vi "Export Config UI.vi"(10 "Config":T1) -> ()   [LabVIEW 2020, in "VolatusGUI.lvlib" / "Historian Charting Manager.lvclass"]
uses:
  Historian Charting Manager.lvclass
  JSON Charting Config.ctl
  JSON Chart Group.ctl
  JSON Plot Group.ctl
  JSON Plot Config.ctl
  Export State.ctl
  lv-tree-tools/Tree Map/Tree Map/Extra Entry Info.ctl
  7dad0396-1ecd-452e-bf08-d6d811beb585.vi
  <vilib>/JDP Science/JSONtext/Variant to JSON Text.vi
  <vilib>/JDP Science/JSONtext/LVClass Serializer/JSONtext LVClass Serializer.lvclass
  Historian Charting Manager.lvclass/Historian Charting Manager.ctl
  lv-tree-tools/Tree Map/Tree Map/Tree Map.lvclass
  VolatusGUI.lvlib
panel:
  in  "Cancel":bool
  in  "Accept":bool
  in  "Plot Groups":string(tree)
  in  "Chart Groups":string(tree)
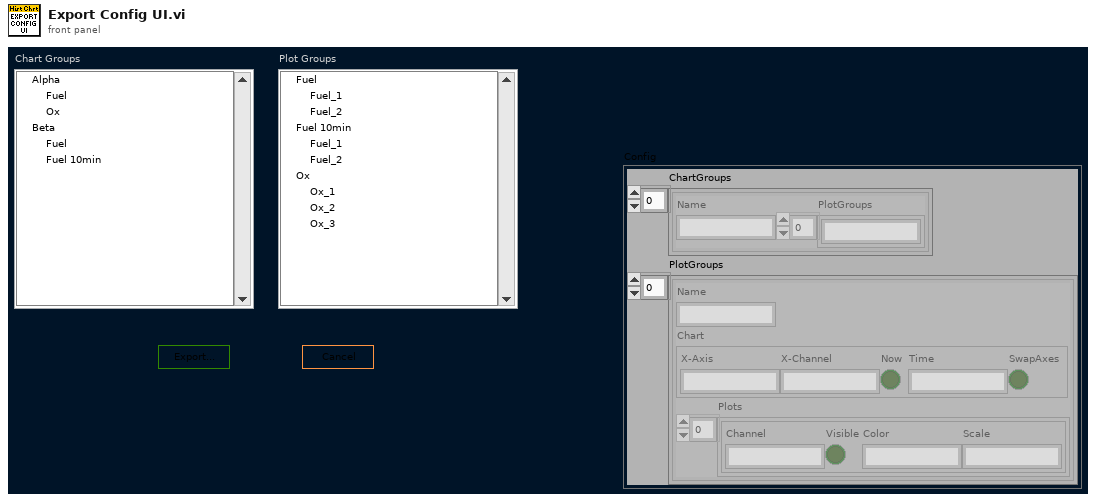
[diagram p1: front panel]
types:
  T1 = typedef "VolatusGUI.lvlib/JSON Charting Config.ctl" = cluster{"ChartGroups":T2[], "PlotGroups":T3[]}
  T2 = typedef "VolatusGUI.lvlib/JSON Chart Group.ctl" = cluster{"Name":string, "PlotGroups":string[]}
  T3 = typedef "VolatusGUI.lvlib/JSON Plot Group.ctl" = cluster{"Name":string, "Chart":cluster{"X-Axis":string, "X-Channel":string, "Now":bool, "Time":string, "SwapAxes":bool}, "Plots":T4[]}
  T4 = typedef "VolatusGUI.lvlib/JSON Plot Config.ctl" = cluster{"Channel":string, "Visible":bool, "Color":string, "Scale":string}
  T5 = typedef "VolatusGUI.lvlib/Historian Charting Manager.lvclass/Export State.ctl" = enum16{"Init", "Select", "Write"}
  T6 = typedef "Tree Map.lvlib/Tree Map.lvclass/Extra Entry Info.ctl" = cluster{"BG Color":u32, "Symbol":i32}
  T7 = enum32{"Invalid", "Standard", "Closed", "Hidden", "Minimized", "Maximized"}
  T8 = typedef "LVPoint32TypeDef.ctl" = cluster{"Horizontal":i32, "Vertical":i32}
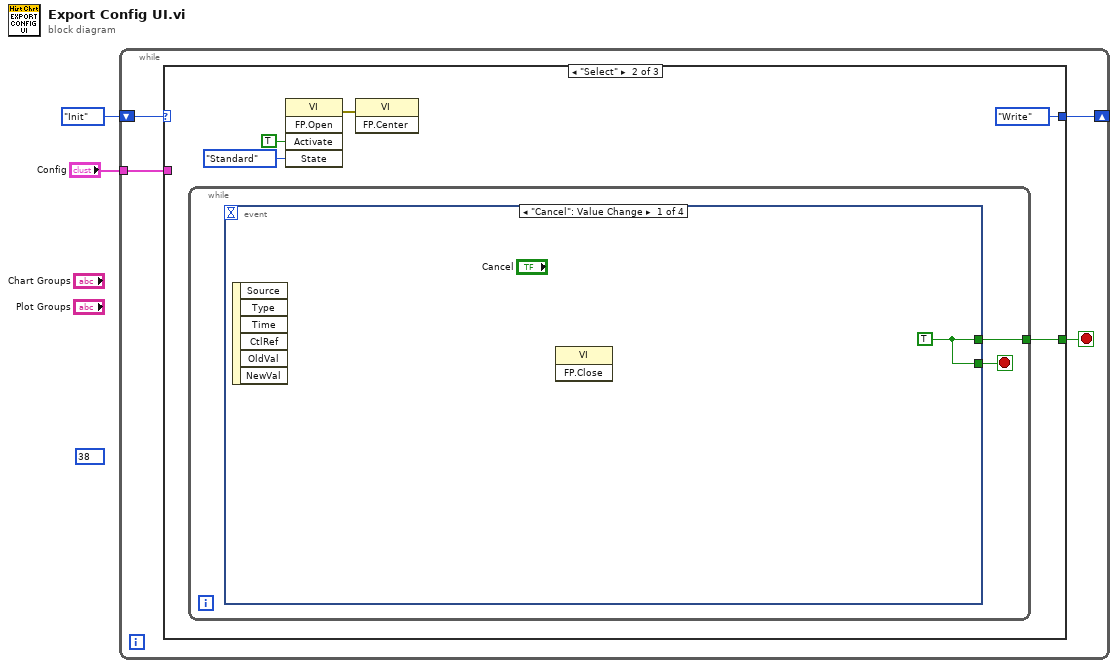
[diagram p0: block diagram]
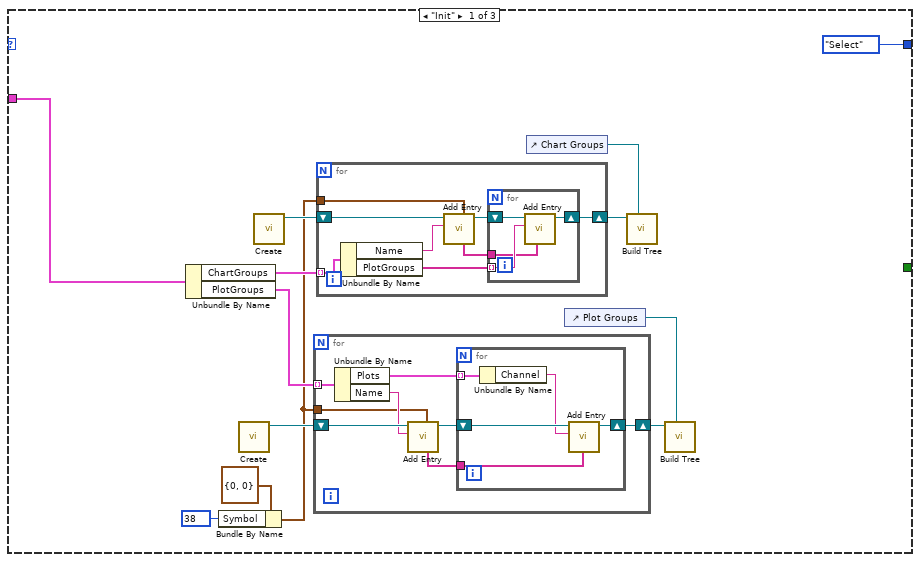
[diagram p2: hidden frame]
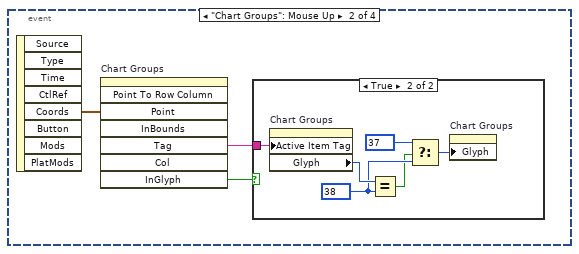
[diagram p3: hidden frame]
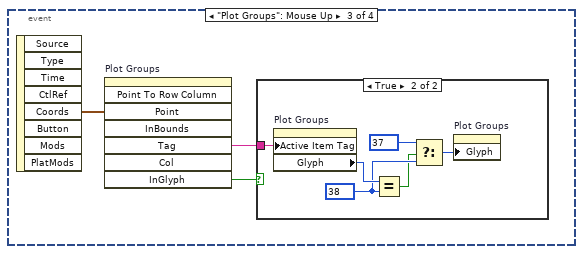
[diagram p5: hidden frame]
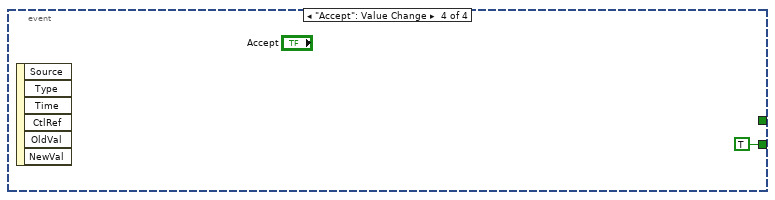
[diagram p7: hidden frame]
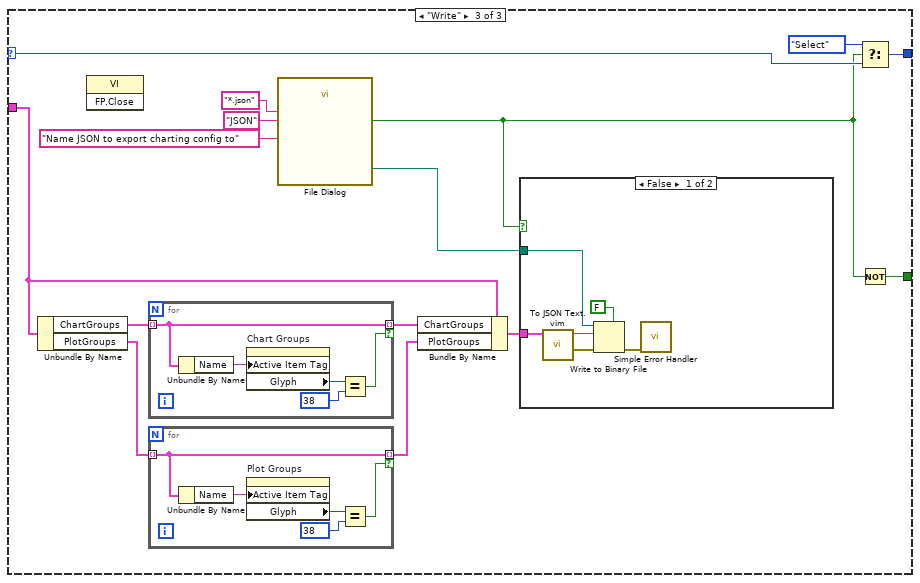
[diagram p8: hidden frame]
diagram:
  (unwired) 38
  n1 = while {
    shift-right: [w5] -> _
    shift-left: Export_State."Init" ("Export State") -> [w6]
    tunnel: "Config" -> [w4]
    stop <- w3 stop-if-true
    n2 = case shown="\"Select\"" w6 {
      selector: w6 -> [_ _ w81]
      tunnel: [Export_State."Select" ("Export State") Export_State."Write" ("Export State") w80] -> w5
      tunnel: w4 -> [w18 _ w74]
      tunnel: [_ w48 w82] -> w3
      frame "Init" {
        n3 = Unbundle By Name(w18) -> ("ChartGroups"=w17:T2[], "PlotGroups"=w13:T3[])
        n4 = Bundle By Name(cluster=T6 {"BG Color"=0, "Symbol"=0} ("Extra Info"), "Symbol"=38) -> (w7:T6)
        n5 = call "Create.vi"() -> ("Tree Map out"=w12:refnum<class "Tree Map.lvclass">)  [unwired: 10 in, 1 out]
        n6 = call "Create.vi"() -> ("Tree Map out"=w16:refnum<class "Tree Map.lvclass">)  [unwired: 10 in, 1 out]
        n7 = for {
          tunnel: w13 -> [w27] mode=indexing
          shift-right: [w21] -> w11
          shift-left: w12 -> [w26]
          tunnel: w7 -> [w20]
          n8 = Unbundle By Name(w27) -> ("Plots"=w23:T4[], "Name"=w25:string)
          n9 = call "Add Entry.vi"("Extra Info"=w20, "Name"=w25, "Tree Map in"=w26) -> ("Tree Map out"=w24:refnum<class "Tree Map.lvclass">, "Hierarchy"=w22:string[])  [unwired: 6 in, 1 out]
          n10 = for {
            shift-right: [w28] -> w21
            shift-left: w24 -> [w31]
            tunnel: w23 -> [w32] mode=indexing
            tunnel: w22 -> [w29]
            n11 = Unbundle By Name(w32) -> ("Channel"=w30:string)
            n12 = call "Add Entry.vi"("Parent (None)"=w29, "Name"=w30, "Tree Map in"=w31) -> ("Tree Map out"=w28:refnum<class "Tree Map.lvclass">)  [unwired: 6 in, 2 out]
          }
        }
        n13 = for {
          tunnel: w17 -> [w40] mode=indexing
          shift-right: [w34] -> w15
          shift-left: w16 -> [w39]
          tunnel: w7 -> [w33]
          n14 = Unbundle By Name(w40) -> ("Name"=w38:string, "PlotGroups"=w36:string[])
          n15 = call "Add Entry.vi"("Extra Info"=w33, "Name"=w38, "Tree Map in"=w39) -> ("Tree Map out"=w37:refnum<class "Tree Map.lvclass">, "Hierarchy"=w35:string[])  [unwired: 6 in, 1 out]
          n16 = for {
            shift-right: [w41] -> w34
            shift-left: w37 -> [w44]
            tunnel: w36 -> [w43] mode=indexing
            tunnel: w35 -> [w42]
            n17 = call "Add Entry.vi"("Parent (None)"=w42, "Name"=w43, "Tree Map in"=w44) -> ("Tree Map out"=w41:refnum<class "Tree Map.lvclass">)  [unwired: 6 in, 2 out]
          }
        }
        n18 = control-ref of="Chart Groups"() -> (w14:refnum<vi>)
        n19 = control-ref of="Plot Groups"() -> (w10:refnum<vi>)
        n20 = call "Build Tree.vi"("Tree"=w14, "Tree Map in"=w15) -> ()  [unwired: 8 in, 2 out]
        n21 = call "Build Tree.vi"("Tree"=w10, "Tree Map in"=w11) -> ()  [unwired: 8 in, 2 out]
      }
      frame "Select" {
        n22 = while {
          tunnel: [w50] -> w48
          stop <- w51 stop-if-true
          n23 = event shown="[0] \"Cancel\": Value Change" {
            selector: _ -> [_ _ _ _]
            dyn-events: _ -> [_ _ _ _]
            timeout: _ -> [_ _ _ _]
            tunnel: [w52 _ _ TRUE] -> w51
            tunnel: [w52 _ _ _] -> w50
            event "Cancel": Value Change {
              w52 = TRUE
              n24 = event-data() -> ()  [unwired: 1 in, 6 out]
              n25 = invoke class="VI" method="FP.Close"() -> ()  [unwired: 3 in, 3 out]
            }
            event "Chart Groups": Mouse Up {
              n26 = event-data() -> ("Coords"=w55:T8)  [unwired: 1 in, 7 out]
              n27 = invoke on="Chart Groups" class="Tree (strict)" method="Point To Row Column"("Point"=w55) -> ("Tag"=w54:string, "InGlyph"=w53:bool)  [unwired: 7 in, 6 out]
              n28 = case shown="True" w53 {
                tunnel: w54 -> [_ w61]
                frame False {
                }
                frame True {
                  w59 = 38
                  n29 = property on="Chart Groups" class="Tree (strict)"("Active Item Tag"=w61) -> ("Glyph"=w60:i32)  [unwired: 2 in, 2 out]
                  n30 = Equal?(x=w60, y=w59) -> (x = y?=w57:bool)
                  n31 = Select(t=37, s=w57, f=w59) -> (s? t:f=w56:i32)
                  n32 = property on="Chart Groups" class="Tree (strict)"("Glyph"=w56) -> ()  [unwired: 2 in, 2 out]
                }
              }
            }
            event "Plot Groups": Mouse Up {
              n33 = event-data() -> ("Coords"=w62:T8)  [unwired: 1 in, 7 out]
              n34 = invoke on="Plot Groups" class="Tree (strict)" method="Point To Row Column"("Point"=w62) -> ("Tag"=w64:string, "InGlyph"=w63:bool)  [unwired: 7 in, 6 out]
              n35 = case shown="True" w63 {
                tunnel: w64 -> [_ w70]
                frame False {
                }
                frame True {
                  w68 = 38
                  n36 = property on="Plot Groups" class="Tree (strict)"("Active Item Tag"=w70) -> ("Glyph"=w69:i32)  [unwired: 2 in, 2 out]
                  n37 = Equal?(x=w69, y=w68) -> (x = y?=w66:bool)
                  n38 = Select(t=37, s=w66, f=w68) -> (s? t:f=w65:i32)
                  n39 = property on="Plot Groups" class="Tree (strict)"("Glyph"=w65) -> ()  [unwired: 2 in, 2 out]
                }
              }
            }
            event "Accept": Value Change {
              n40 = event-data() -> ()  [unwired: 1 in, 6 out]
            }
          }
        }
        n41 = invoke class="VI" method="FP.Open"("Activate"=TRUE ("Activate?"), "State"=T7."Standard") -> (error out=w47:errorcluster)  [unwired: 3 in, 4 out]
        n42 = invoke class="VI" method="FP.Center"(error in=w47) -> ()  [unwired: 2 in, 3 out]
      }
      frame "Write" {
        n43 = Unbundle By Name(w74) -> ("ChartGroups"=w79:T2[], "PlotGroups"=w77:T3[])
        n44 = invoke class="VI" method="FP.Close"() -> ()  [unwired: 3 in, 3 out]
        n45 = for {
          tunnel: w79 -> [w101] mode=indexing
          tunnel: [w101] -> w78 mode=indexing if=w98
          n46 = Unbundle By Name(w101) -> ("Name"=w102:string)
          n47 = property on="Chart Groups" class="Tree (strict)"("Active Item Tag"=w102) -> ("Glyph"=w100:i32)  [unwired: 2 in, 2 out]
          n48 = Equal?(x=w100, y=38) -> (x = y?=w98:bool)
        }
        n49 = for {
          tunnel: w77 -> [w96] mode=indexing
          tunnel: [w96] -> w76 mode=indexing if=w93
          n50 = Unbundle By Name(w96) -> ("Name"=w97:string)
          n51 = property on="Plot Groups" class="Tree (strict)"("Active Item Tag"=w97) -> ("Glyph"=w95:i32)  [unwired: 2 in, 2 out]
          n52 = Equal?(x=w95, y=38) -> (x = y?=w93:bool)
        }
        n53 = call "File Dialog"("prompt"="Name JSON to export charting config to", "pattern (all files)"="*.json", "pattern label"="JSON") -> ("selected path"=w72:path, "cancelled"=w73:bool)  [unwired: 9 in, 2 out]
        n54 = Bundle By Name(cluster=w74, "ChartGroups"=w78, "PlotGroups"=w76) -> (w75:T1)
        n55 = case shown="False" w73 {
          tunnel: w75 -> [w92 _]
          tunnel: w72 -> [w88 _]
          frame False {
            n56 = call "To JSON Text.vim"("Anything"=w92) -> ("error out"=w91:errorcluster, "<JSON>"=w90:string)  [unwired: 9 in]
            n57 = Write to Binary File(file (use dialog)=w88, data=w90, error in=w91, 5:FALSE ("prepend array or string size? (T)")) -> (error out=w87:errorcluster)  [unwired: 2 in, 2 out]
            n58 = call <vilib>:"Simple Error Handler.vi"("error in (no error)"=w87) -> ()  [unwired: 4 in, 5 out]
          }
          frame True {
          }
        }
        n59 = Select(t=Export_State."Select" ("Export State"), s=w73, f=w81) -> (s? t:f=w80:T5)
        n60 = Not(x=w73) -> (.not. x?=w82:bool)
      }
    }
  }
